vi "Sys config window-Update config.vi"() -> (0 "error out":errorcluster)   [LabVIEW 2017]
uses:
  Typedefs/HW config states enum.ctl
  Visualisation/Functional Imaging Viewer/Typedefs/Get-Set-Clear Control.ctl
  Configuration code/Calibration/Globals/gl_Calibration globals.vi
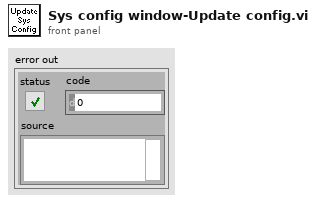
[diagram p1: front panel]
types:
  T1 = typedef "Get-Set-Clear Control.ctl" = enum16{"Get", "Set", "Clear"}
  T2 = typedef "HW config states enum.ctl" = enum16{"Load from file", "Save to file", "Write all", "Read all", "Write XY stage settings", "Write DAQ FPGA settings", "Write Control FPGA settings", "Write Phys Channels", "Write System Config", "Write HW Config", "Save System Config", "Save HW Config", "Clear", "Compare from file"}
  T3 = typedef "Initial config.ctl" = cluster{"Triggers output setup":T4, "General trigger settings":T6, "Calibration settings":T8, "Hardware Configuration":T9, "System Config":T24, "Calibration config.":T27, "General Setup":T31, "AOD Settings - distilled":T32}
  T4 = typedef "Triggers output setup.ctl" = T5[]
  T5 = typedef "Trigger setup element cluster.ctl" = cluster{"Name":string, "Output?":bool, "Output terminal":tag, "PXI backplane line":tag, "Pulse width (us)":u16}
  T6 = typedef "General trigger settings cluster.ctl" = cluster{"Trigger 1 function":T7, "Triggers loop clock (MHz)":dbl}
  T7 = typedef "Trigger 1 selector enum.ctl" = enum16{"Encoder trigger", "Line trigger", "Control system's ref frame acknowledgement"}
  T8 = typedef "Pockels Calibration settings cluster.ctl" = cluster{"Pockels cal.Zoom":u8, "Pockels cal.Dwell time (µs)":dbl}
  T9 = typedef "Hardware Configuration settings.ctl" = cluster{"Dev. PC":bool, "Swap XY on stage":bool, "No of AOD":u8, "MC Supported":bool, "Axial MC":bool, "Computer MAC address":string, "Externalise Triggers":bool, "Trigger HW config":T10, "DAQmx Chan":T11, "XY stage available":bool, "XY Stage":T12, "Z stage available":bool, "Z Stage config cluster":T13, "Encoder available":bool, "Encoder":T14, "VidRec available":bool, "Cam VidRec":T15, "Laser Power Control HW config":T16, "Laser 1 available":bool, "Laser 1 config cluster":T17, "Prechirper 1 available":bool, "Prechirper 1 config cluster":T18, "Control system.FPGA available?":bool, "Control Sys. HW config":T19, "DAQ FPGA HW Config":T20}
  T10 = typedef "Triggers HW config.ctl" = cluster{"Available Device List":i32, "Device Address":string}
  T11 = typedef "DAQmx physical channels cluster.ctl" = cluster{"Pockels AO":tag, "Hard shutter AO":tag, "PMT AOs":tag, "Galvo AOs":tag, "Power meter AI":tag}
  T12 = typedef "XY Stage config cluster.ctl" = cluster{"COM port":refnum<visa-resource-name>, "XY stage available":bool, "Baudrate":i32, "Type":string}
  T13 = typedef "Z Stage config cluster.ctl" = cluster{"COM port":refnum<visa-resource-name>, "Z stage available":bool, "Baudrate":i32, "Type":string}
  T14 = typedef "Encoder config cluster.ctl" = cluster{"IP address":string, "Port":u16, "Encoder available":bool, "Wheel radius (cm)":dbl, "Encoder Trigger":tag}
  T15 = typedef "Cam VidRec HW config setup cluster.ctl" = cluster{"DO flag-Video record":tag, "DO flag-Trial start":tag, "VidRec available":bool}
  T16 = typedef "Laser Power Control HW config.ctl" = cluster{"Laser Power Control":string, "Laser Power Modulation Control":enum16{"NI", "FPGA"}}
  T17 = typedef "Laser 1 config cluster.ctl" = cluster{"COM port":refnum<visa-resource-name>, "Laser 1 available":bool, "Baud Rate":i32, "Type":string}
  T18 = typedef "PreChirper 1 config cluster.ctl" = cluster{"Type":string, "Baud Rate":i32, "Prechirper 1 available":bool, "COM port":refnum<visa-resource-name>}
  T19 = typedef "Control Sys HW config cluster.ctl" = cluster{"Control system.FPGA available?":bool, "Control system.FPGA Type":enum16{"Virtex 5", "Virtex 7"}, "Control system.Network adapter name":string, "Control system.MAC address":string, "Control system.Ethernet Port":u32, "Control system.Ethernet Port Opened":bool}
  T20 = typedef "DAQ FPGA HW config cluster.ctl" = cluster{"FGPA Ref":T21, "Target":T22, "input card type":T23}
  T21 = typedef "FPGA Ref.ctl" = refnum<k20>
  T22 = typedef "nirio_resource_hc.ctl" = tag
  T23 = typedef "FPGA input type AC-DC.ctl" = enum16{"AC Card", "DC Card"}
  T24 = typedef "System Configuration.ctl" = cluster{"Laser wavelength (nm)":dbl, "DAQ FPGA System":T25, "Control system":T26}
  T25 = typedef "DAQ FPGA system config.ctl" = cluster{"Clock Freq (MHz) ":dbl, "Samples Wait after Trigger":u16, "AOD fill":u16, "StartupDelay":i32, "Slip Cycle (clock cycles)":u32, "Add Cycle":bool}
  T26 = typedef "CTRL system config.ctl" = cluster{"AOD 1 Amplitude":i16, "AOD 2 Amplitude":i16, "AOD 3 Amplitude":i16, "AOD 4 Amplitude":i16, "AOD 5 Amplitude":i16, "AOD 6 Amplitude":i16, "T0 (ns)":dbl, "Ta (ns)":dbl, "Data Time Interval (ns)":dbl, "Ctrl FPGA Clock (MHz)":dbl}
  T27 = typedef "Calibration config.ctl" = cluster{"Current Objective":string, "Objective Settings":T28[], "PreChirper Values Preset ?":bool, "PreChirper Settings":T29[], "PreChirper Constants":T30}
  T28 = typedef "Objective Config.ctl" = cluster{"Name":string, "Sum X":dbl, "Sum Y":dbl, "Diff X":dbl, "Diff Y":dbl, "Distortion Correction":dbl, "Z_norm to um_scaling":dbl, "X_norm to um_scaling":dbl, "Calibrated Wavelength":dbl}
  T29 = typedef "Prechirper Cal Config.ctl" = cluster{"Wavelength":i32, "Prism 1":i32, "Prism 2":i32}
  T30 = typedef "PreChirper constants.ctl" = cluster{"a 1":i32, "b 1":i32, "c 1":i32, "a 2":i32, "b 2":i32, "c 2":i32, "lmin":i32, "lmax":i32}
  T31 = typedef "General Setup.ctl" = cluster{"Microscope ID":string, "Microscope Type":string, "Revision Number":string, "Advanced Imaging":bool, "Error Logging":bool, "Performance Monitoring":bool, "Max Allowed Trial Length":dbl, "Initial Scan Resolution":dbl, "Initial Acceptance Angle":dbl, "Initial Laser Wavelength":dbl, "Initial Dwell Time":dbl}
  T32 = typedef "AOD Settings-distilled.ctl" = cluster{"AOD 1 thickness (mm)":dbl, "AOD 2 thickness (mm)":dbl, "AOD 3 thickness (mm)":dbl, "AOD 4 thickness (mm)":dbl, "AOD 1-2 separation (mm)":dbl, "AOD 2-3 separation (mm)":dbl, "AOD 3-4 separation (mm)":dbl, "AOD 1 Centre (mm)":dbl, "AOD 2 Centre (mm)":dbl, "AOD 3 Centre (mm)":dbl, "AOD 4 Centre (mm)":dbl, "AOD 1 X Offset":dbl, "AOD 2 X Offset":dbl, "AOD 3 X Offset":dbl, "AOD 4 X Offset":dbl, "AOD 1 Y Offset":dbl, "AOD 2 Y Offset":dbl, "AOD 3 Y Offset":dbl, "AOD 4 Y Offset":dbl, "Timing Offset AOD 1":dbl, "Timing Offset AOD 2":dbl, "Timing Offset AOD 3":dbl, "Timing Offset AOD 4":dbl, "AOL centre wavelength (nm)":dbl, "AOL centre frequency (MHz)":dbl, "Pair deflection ratio":dbl, "AOL aperture (mm)":dbl, "AOD fill time (us)":dbl, "Diffraction mode":dbl, "Crystal length (mm)":dbl, "Acoustic velocity (m/s)":dbl, "AOD Ord. Refractive index":dbl}
  T33 = typedef "AOL Properties Cluster.ctl" = cluster{"AOD 1 thickness (mm)":dbl, "AOD 2 thickness (mm)":dbl, "AOD 3 thickness (mm)":dbl, "AOD 4 thickness (mm)":dbl, "AOD 5 thickness (mm)":dbl, "AOD 6 thickness (mm)":dbl, "AOD 1-2 separation (mm)":dbl, "AOD 2-3 separation (mm)":dbl, "AOD 3-4 separation (mm)":dbl, "AOD 4-5 separation (mm)":dbl, "AOD 5-6 separation (mm)":dbl, "AOD 1 X Offset":dbl, "AOD 2 X Offset":dbl, "AOD 3 X Offset":dbl, "AOD 4 X Offset":dbl, "AOD 1 Y Offset":dbl, "AOD 2 Y Offset":dbl, "AOD 3 Y Offset":dbl, "AOD 4 Y Offset":dbl, "AOD 1 X Direction":dbl, "AOD 2 X Direction":dbl, "AOD 3 X Direction":dbl, "AOD 4 X Direction":dbl, "AOD 1 Y Direction":dbl, "AOD 2 Y Direction":dbl, "AOD 3 Y Direction":dbl, "AOD 4 Y Direction":dbl, "AOD 1 Centre (mm)":dbl, "AOD 2 Centre (mm)":dbl, "AOD 3 Centre (mm)":dbl, "AOD 4 Centre (mm)":dbl, "Timing Offset AOD 1":dbl, "Timing Offset AOD 2":dbl, "Timing Offset AOD 3":dbl, "Timing Offset AOD 4":dbl, "AOD Optical offset 1":dbl, "AOD Optical offset 2":dbl, "AOL aperture (mm)":dbl, "AOL centre wavelength (nm)":dbl, "AOL centre frequency (MHz)":dbl, "Diffraction mode":dbl, "Crystal length (mm)":dbl, "Acoustic velocity (m/s)":dbl, "Pair deflection ratio":dbl, "AOD fill time (us)":dbl, "AOD Ord. Refractive index":dbl, "AOD ExtraOrd. Refractive index":dbl}
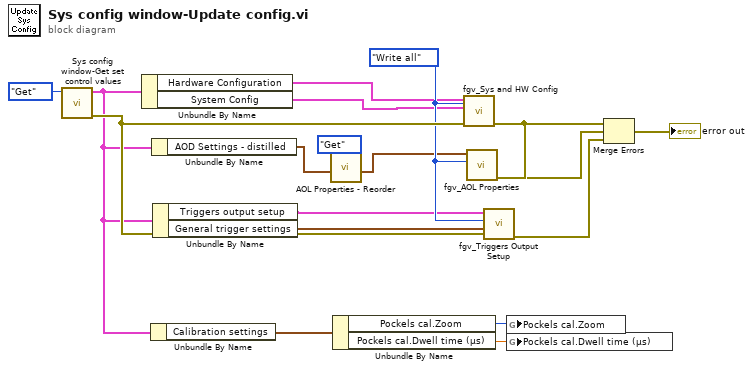
[diagram p0: block diagram]
diagram:
  w16 = HW_config_states_enum."Write all" ("Function")
  n1 = call "Sys config window-Get set control values.vi"("Function"=Get-Set-Clear_Control."Get") -> ("error out"=w17:errorcluster, "output cluster"=w7:T3)  [unwired: 9 in]
  n2 = Unbundle By Name(w7) -> ("Hardware Configuration"=w8:T9, "System Config"=w9:T24)
  n3 = Unbundle By Name(w7) -> ("Calibration settings"=w13:T8)
  n4 = Unbundle By Name(w7) -> ("AOD Settings - distilled"=w5:T32)
  n5 = Unbundle By Name(w7) -> ("Triggers output setup"=w14:T4, "General trigger settings"=w10:T6)
  n6 = call "AOL Properties - Reorder.vi"("Function"=Get-Set-Clear_Control."Get", "Value"=w5) -> ("AOL Properties out"=w4:T33)  [unwired: 8 in, 1 out]
  n7 = Unbundle By Name(w13) -> ("Pockels cal.Zoom"=w12:u8, "Pockels cal.Dwell time (µs)"=w11:dbl)
  n8 = call "fgv_Sys and HW Config.vi"("Function"=w16, "error in (no error)"=w17, "System Config"=w9, "Hardware Configuration"=w8) -> ("error out"=w2:errorcluster)  [unwired: 5 in, 2 out]
  n9 = call "fgv_AOL Properties.vi"("error in (no error)"=w2, "Function"=w16, "AOL Properties in"=w4) -> ("error out"=w1:errorcluster)  [unwired: 7 in, 1 out]
  n10 = call "fgv_Triggers Output Setup.vi"("error in (no error)"=w17, "General trigger settings"=w10, "Function"=w16, "Triggers output setup"=w14) -> ("error out"=w3:errorcluster)  [unwired: 5 in, 2 out]
  n11 = global write "gl_Calibration globals.vi" "Pockels cal.Zoom"(w12) -> ()
  n12 = global write "gl_Calibration globals.vi" "Pockels cal.Dwell time (µs)"(w11) -> ()
  n13 = Merge Errors(w2, w1, w3) -> (→"error out":errorcluster)
